vi "MaxiumCentered.vi"(11 "Input Y Values":dbl[](array[numeric])) -> (2 "State output":T1(ring), 3 "Output Y Values":dbl[](array[numeric]))   [LabVIEW 2014]
panel:
  in  "Input Location of Trigger":dbl
  # "CenterMax VI"
  # "Is the Waveform Trigger in the Middle?"
  # "Inputs"
  # "Outputs"
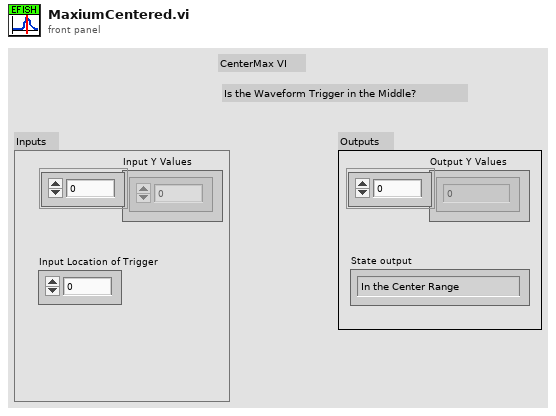
[diagram p1: front panel]
types:
  T1 = enum16{"In the Center Range", "Before the Center Range", "After the Center Range"}
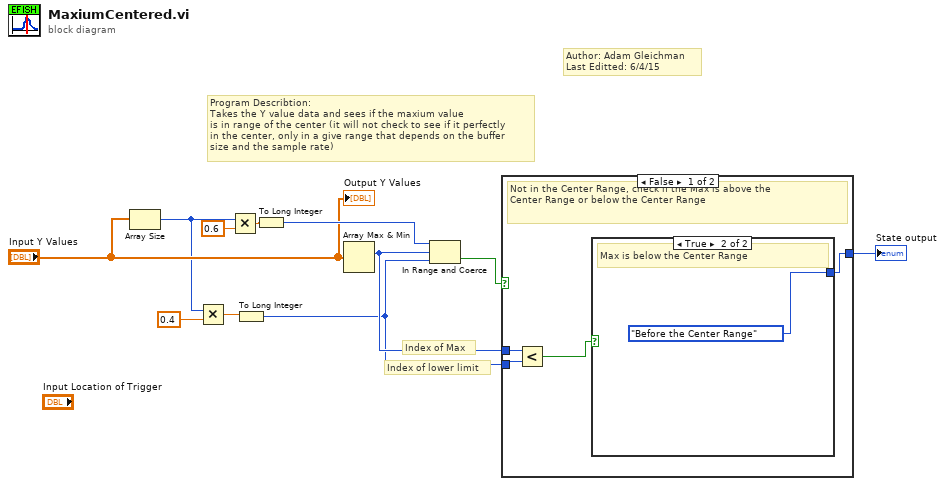
[diagram p0: block diagram]
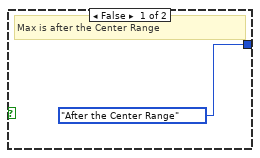
[diagram p2: hidden frame]
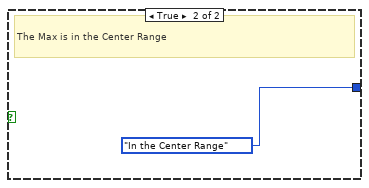
[diagram p3: hidden frame]
diagram:
  # "Index of lower limit"
  # "Index of Max"
  # "Program Describtion: \nTakes the Y value data and sees if the maxium value\nis in range of the center (it will not check to see if it perfectly\nin the center, only in a give range that depends on the buffer\nsize and the sample rate)"
  # "Author: Adam Gleichman\nLast Editted: 6/4/15"
  n1 = Array Size(array="Input Y Values") -> (size(s)=w1:i32)
  n2 = Multiply(x=w1, y=0.4) -> (x*y=w5:dbl)
  n3 = Multiply(x=w1, y=0.6) -> (x*y=w6:dbl)
  n4 = To Long Integer(number=w5) -> (32bit integer=w4:i32)
  n5 = To Long Integer(number=w6) -> (32bit integer=w3:i32)
  n6 = Array Max & Min(array="Input Y Values") -> (max index (indices)=w8:i32)  [unwired: 3 out]
  n7 = In Range and Coerce(upper limit=w3, x=w8, lower limit=w4) -> (In Range?=w10:bool)  [unwired: 1 out]
  n8 = case shown="False" w10 {
    tunnel: [w12 T1."In the Center Range" ("something")] -> w9
    tunnel: w4 -> [w14 _]
    tunnel: w8 -> [w15 _]
    frame False {
      # "Not in the Center Range, check if the Max is above the \nCenter Range or below the Center Range"
      n9 = Less?(x=w15, y=w14) -> (x < y?=w13:bool)
      n10 = case shown="True" w13 {
        tunnel: [T1."After the Center Range" ("something") T1."Before the Center Range" ("something")] -> w12
        frame False {
          # "Max is after the Center Range"
        }
        frame True {
          # "Max is below the Center Range"
        }
      }
    }
    frame True {
      # "The Max is in the Center Range"
    }
  }
  "State output" <- w9
  "Output Y Values" <- "Input Y Values"
